vi "Fill Out Unref Files.vi"(7 "Unreferenced Files":path[](array[path]), 8 "error in (no error)":errorcluster, 11 "NI_report in":refnum<class "NI_report.lvclass">) -> (0 "error out":errorcluster, 3 "NI_report out":refnum<class "NI_report.lvclass">)   [LabVIEW 2014]
uses:
  <vilib>/Utility/NIReport.llb/NI_report.lvclass
  <vilib>/addons/_office/excel.llb/Excel Easy Table (str).vi
  <vilib>/Utility/NIReport.llb/Excel/NI_Excel.lvclass
  <vilib>/addons/_office/NI_ReportGenerationToolkit.lvlib
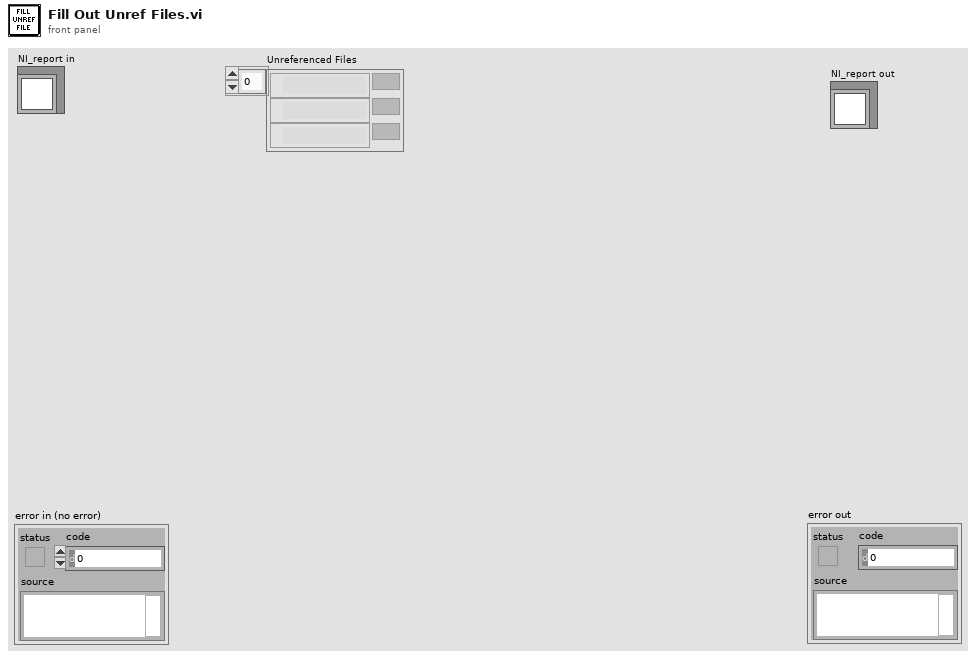
[diagram p1: front panel]
types:
  T1 = cluster{"on/off":bool, "weight":i32, "color":u32}
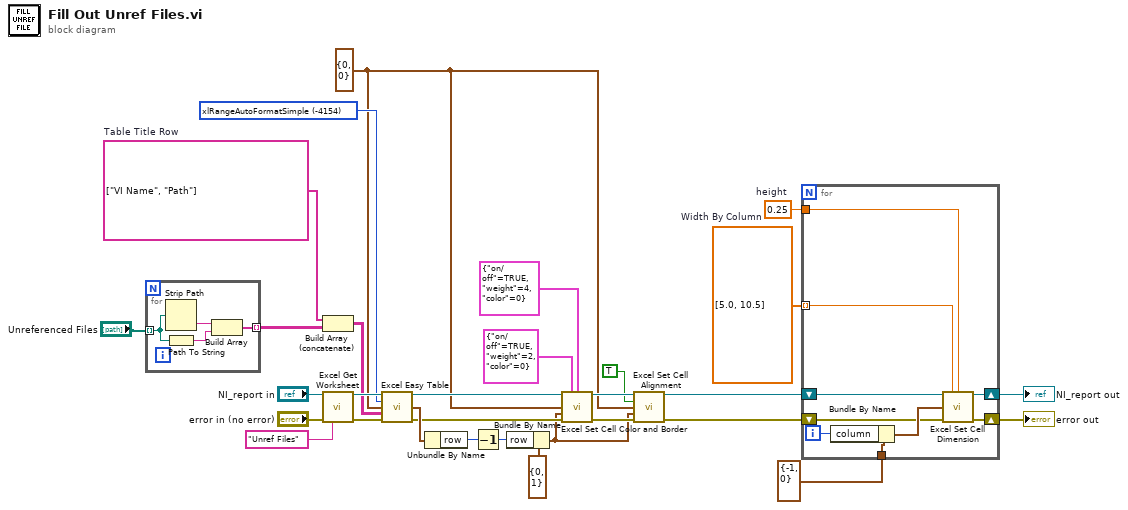
[diagram p0: block diagram]
diagram:
  w10 = 0.25  # height
  w15 = dbl[] [5.0, 10.5]  # Width By Column
  w21 = string[] ["VI Name", "Path"]  # Table Title Row
  w22 = -4154 items=["xlRangeAutoFormat3DEffects1"=13, "xlRangeAutoFormat3DEffects2"=14, "xlRangeAutoFormatAccounting1"=4, "xlRangeAutoFormatAccounting2"=5, "xlRangeAutoFormatAccounting3"=6, "xlRangeAutoFormatAccounting4"=17, "xlRangeAutoFormatClassic1"=1, "xlRangeAutoFormatClassic2"=2, "xlRangeAutoFormatClassic3"=3, "xlRangeAutoFormatColor1"=7, "xlRangeAutoFormatColor2"=8, "xlRangeAutoFormatColor3"=9, "xlRangeAutoFormatList1"=10, "xlRangeAutoFormatList2"=11, "xlRangeAutoFormatList3"=12, "xlRangeAutoFormatLocalFormat1"=15, "xlRangeAutoFormatLocalFormat2"=16, "xlRangeAutoFormatLocalFormat3"=19, "xlRangeAutoFormatLocalFormat4"=20, "xlRangeAutoFormatReport1"=21, "xlRangeAutoFormatReport2"=22, "xlRangeAutoFormatReport3"=23, "xlRangeAutoFormatReport4"=24, "xlRangeAutoFormatReport5"=25, "xlRangeAutoFormatReport6"=26, "xlRangeAutoFormatReport7"=27, "xlRangeAutoFormatReport8"=28, "xlRangeAutoFormatReport9"=29, "xlRangeAutoFormatReport10"=30, "xlRangeAutoFormatClassicPivotTable"=31, "xlRangeAutoFormatTable1"=32, "xlRangeAutoFormatTable2"=33, "xlRangeAutoFormatTable3"=34, "xlRangeAutoFormatTable4"=35, "xlRangeAutoFormatTable5"=36, "xlRangeAutoFormatTable6"=37, "xlRangeAutoFormatTable7"=38, "xlRangeAutoFormatTable8"=39, "xlRangeAutoFormatTable9"=40, "xlRangeAutoFormatTable10"=41, "xlRangeAutoFormatPTNone"=42, "xlRangeAutoFormatNone"=-4142, "xlRangeAutoFormatSimple"=-4154] ("auto format (none)")
  w14 = cluster{"row":i32, "column":i32} {"row"=0, "column"=0} ("start (-1, -1)")
  n1 = for {
    tunnel: "Unreferenced Files" -> [w34] mode=indexing
    tunnel: [w31] -> w1 mode=indexing
    n2 = Strip Path(path=w34) -> (name=w33:string)  [unwired: 1 out]
    n3 = Path To String(path=w34) -> (string=w32:string)
    n4 = Build Array(w33, w32) -> (w31:string[])
  }
  n5 = Build Array (concatenate)(w21, w1) -> (w20:string[][])
  n6 = call <vilib>:"Excel Get Worksheet.vi"("report in"="NI_report in", "error in (no error)"="error in (no error)", "name (\"\")"="Unref Files" ("name (\"\")")) -> ("report out"=w27:refnum<class "NI_report.lvclass">, "error out"=w28:errorcluster)  [unwired: 11 in]
  n7 = call-poly <vilib>:"Excel Easy Table.vi"("report in"=w27, "auto format (none)"=w22, "start (0, 0)"=w14, "text data"=w20, "error in (no error)"=w28) -> ("report out"=w25:refnum<class "NI_report.lvclass">, "next cell bottom-left"=w18:cluster{"row":i32, "column":i32}, "error out"=w12:errorcluster)  [unwired: 6 in, 2 out]
  n8 = Unbundle By Name(w18) -> ("row"=w5:i32)
  n9 = Decrement(x=w5) -> (x-1=w17:i32)
  n10 = Bundle By Name(cluster=cluster{"row":i32, "column":i32} {"row"=0, "column"=1} ("start (-1, -1)"), "row"=w17) -> (w7:cluster{"row":i32, "column":i32})
  n11 = call <vilib>:"Excel Set Cell Color and Border.vi"("report in"=w25, "inside border"=T1 {"on/off"=TRUE, "weight"=2, "color"=0}, "outside border"=T1 {"on/off"=TRUE, "weight"=4, "color"=0}, "start (-1, -1)"=w14, "end (-1, -1)"=w7, "error in (no error)"=w12) -> ("report out"=w19:refnum<class "NI_report.lvclass">, "error out"=w11:errorcluster)  [unwired: 8 in]
  n12 = call <vilib>:"Excel Set Cell Alignment.vi"("report in"=w19, "wrap text? (F)"=TRUE, "start (-1, -1)"=w14, "end (-1, -1)"=w7, "error in (no error)"=w11) -> ("report out"=w9:refnum<class "NI_report.lvclass">, "error out"=w8:errorcluster)  [unwired: 9 in]
  n13 = for {
    tunnel: w15 -> [w41] mode=indexing
    tunnel: cluster{"row":i32, "column":i32} {"row"=-1, "column"=0} ("start (-1, -1)") -> [w40]
    shift-right: [w42] -> w4
    shift-left: w9 -> [w43]
    shift-right: [w39] -> w3
    shift-left: w8 -> [w36]
    tunnel: w10 -> [w35]
    i -> [w37]
    n14 = Bundle By Name(cluster=w40, "column"=w37) -> (w38:cluster{"row":i32, "column":i32})
    n15 = call <vilib>:"Excel Set Cell Dimension.vi"("report in"=w43, "width (-1)"=w41, "height (-1)"=w35, "start (-1, -1)"=w38, "error in (no error)"=w36) -> ("report out"=w42:refnum<class "NI_report.lvclass">, "error out"=w39:errorcluster)  [unwired: 9 in]
  }
  "error out" <- w3
  "NI_report out" <- w4
